vi "Task Return.vi"(8 "error in (no error)":errorcluster, 10 "Queue Time Out  (ms)":u32=3000, 11 "Self Addressed Task in":refnum<class "Self Addressed Task.lvclass">) -> (0 "error out":errorcluster, 1 "Success":bool, 2 "Task Out":refnum<class "Task Ancestor.lvclass">, 3 "Self Addressed Task out":refnum<class "Self Addressed Task.lvclass">)   [LabVIEW 2024, in "Self Addressed Task.lvclass"]
uses:
  Self Addressed Task.lvclass
  Self Addressed Task.lvclass/Self Addressed Task.ctl
  Task Ancestor/Task Ancestor.lvclass
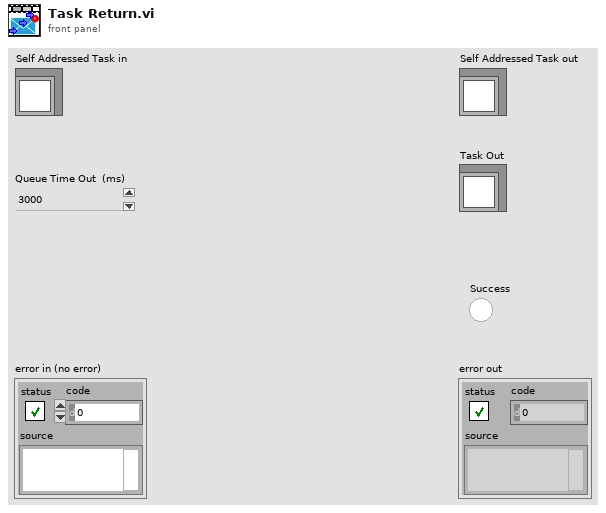
[diagram p1: front panel]
types:
  T1 = typedef "Return Address.ctl" = refnum<queue>
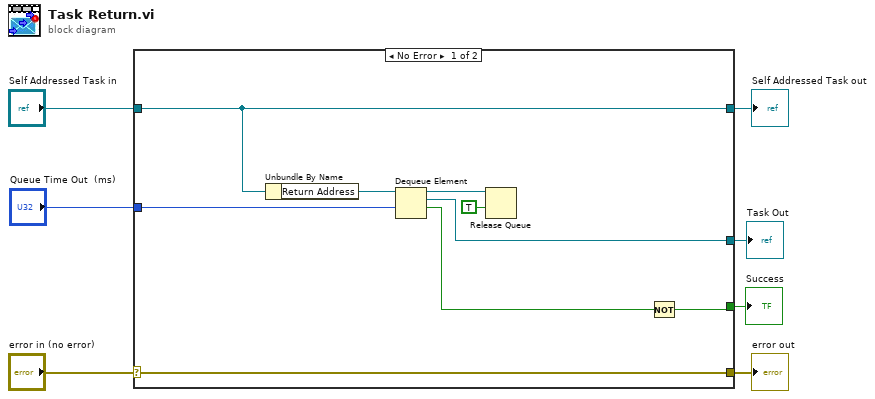
[diagram p0: block diagram]
diagram:
  n1 = case shown="No Error" "error in (no error)" {
    selector: "error in (no error)" -> [w16 w18]
    tunnel: [w16 w18] -> w6
    tunnel: [w15 w17] -> w4
    tunnel: "Self Addressed Task in" -> [w15 w17]
    tunnel: "Queue Time Out  (ms)" -> [w13 _]
    tunnel: [w10 _] -> w2
    tunnel: [w9 _] -> w1
    frame No Error {
      n2 = Unbundle By Name(w15) -> ("Return Address"=w14:T1)
      n3 = Dequeue Element(queue=w14, timeout in ms (-1)=w13) -> (queue out=w12:T1, element=w10:refnum<class "Task Ancestor.lvclass">, timed out?=w8:bool)  [unwired: 1 in, 1 out]
      n4 = Release Queue(queue=w12, force destroy? (F)=TRUE) -> ()  [unwired: 1 in, 3 out]
      n5 = Not(x=w8) -> (.not. x?=w9:bool)
    }
    frame Error {
    }
  }
  "error out" <- w6
  "Self Addressed Task out" <- w4
  "Task Out" <- w2
  "Success" <- w1
